vi "FTW-Endpoint-Multipart-Ask.vi"(0 "FTW Endpoint":refnum<class "FTW-Endpoint-Notifier.lvclass">, 5 "Multipart Message":string[](array[string]), 7 "Read Timeout":i32=100 format="%dmsec", 9 "Write Timeout":i32 format="%dmsec", 11 "error in":errorcluster) -> (4 "FTW Endpoint out":refnum<class "FTW-Endpoint-Notifier.lvclass">, 6 "Reply":string[](array[string]), 8 "Read Timed out?":bool, 10 "Write Timed out?":bool, 15 "error out":errorcluster)   [LabVIEW 2013, in "FTW-Endpoint-Notifier.lvclass"]
uses:
  FTW-Endpoint-Notifier.lvclass
  FTW-Endpoint-Notifier.lvclass/FTW-Endpoint-Notifier.ctl
  Endpoint/FTW-Endpoint.lvclass
  Ether/FTW-Ether.lvclass
panel:
  # "Inputs"
  # "Outputs"
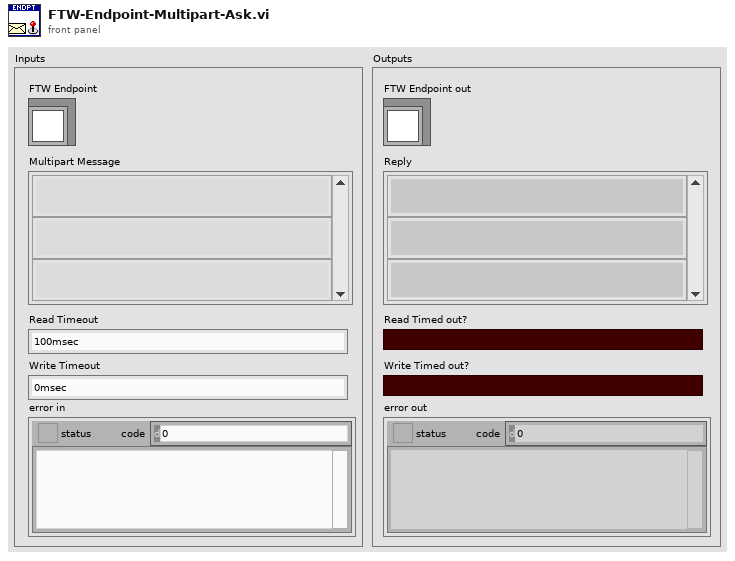
[diagram p1: front panel]
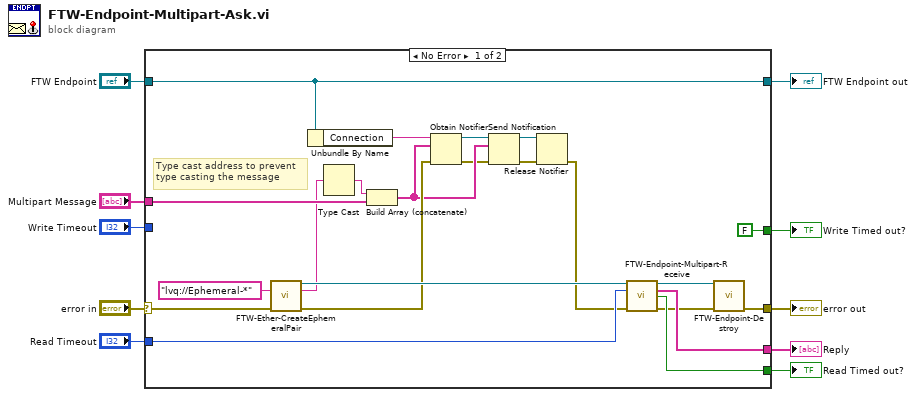
[diagram p0: block diagram]
diagram:
  n1 = case shown="No Error" "error in" {
    selector: "error in" -> [w31 w34]
    tunnel: [w24 w34] -> w10
    tunnel: [w20 w33] -> w8
    tunnel: "FTW Endpoint" -> [w20 w33]
    tunnel: "Multipart Message" -> [w32 _]
    tunnel: "Read Timeout" -> [w29 _]
    tunnel: [w27 _] -> w4
    tunnel: [w28 _] -> w3
    tunnel: [FALSE _] -> w2
    tunnel: "Write Timeout" -> [_ _]
    frame No Error {
      # "Type cast address to prevent\ntype casting the message"
      n2 = call "FTW-Ether-CreateEphemeralPair.vi"("Requested Ephemeral Address"="lvq://Ephemeral-*", "error in"=w31) -> ("Ephemeral Endpoint"=w30:refnum<class "FTW-Endpoint.lvclass">, "Actual Ephemeral Address"=w15:string, "error out"=w22:errorcluster)  [unwired: 11 in]
      n3 = Unbundle By Name(w20) -> ("Connection"=w17:string)
      n4 = Type Cast(x=w15) -> (*(type *) &x=w14:string)  [unwired: 1 in]
      n5 = Build Array (concatenate)(w14, w32) -> (w19:string[])
      n6 = Obtain Notifier(name (unnamed)=w17, notification data type=w19, error in (no error)=w22) -> (notifier out=w18:refnum<notifier>, error out=w13:errorcluster)  [unwired: 1 in, 1 out]
      n7 = Send Notification(notification=w19, notifier=w18, error in (no error)=w13) -> (notifier out=w16:refnum<notifier>, error out=w12:errorcluster)
      n8 = Release Notifier(notifier=w16, error in (no error)=w12) -> (error out=w21:errorcluster)  [unwired: 1 in, 2 out]
      n9 = call-dynamic "FTW-Endpoint-Multipart-Receive.vi"("FTW Endpoint"=w30, "Timeout"=w29, "error in"=w21) -> ("FTW Endpoint out"=w26:refnum<class "FTW-Endpoint.lvclass">, "Message Received"=w28:string[], "Timed out?"=w27:bool, "error out"=w25:errorcluster)  [unwired: 9 in]
      n10 = call-dynamic "FTW-Endpoint-Destroy.vi"("FTW Endpoint"=w26, "error in"=w25) -> ("error out"=w24:errorcluster)  [unwired: 13 in]
    }
    frame Error {
    }
  }
  "error out" <- w10
  "FTW Endpoint out" <- w8
  "Read Timed out?" <- w4
  "Reply" <- w3
  "Write Timed out?" <- w2
